vi "New GUID.vi"(8 "error in (no error)":errorcluster) -> (0 "error out":errorcluster, 2 "GUID bytes":u8[](array[numeric]) format="%02x", 3 "GUID":string)   [LabVIEW 2013]
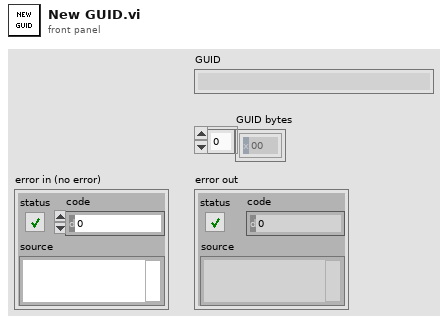
[diagram p1: front panel]
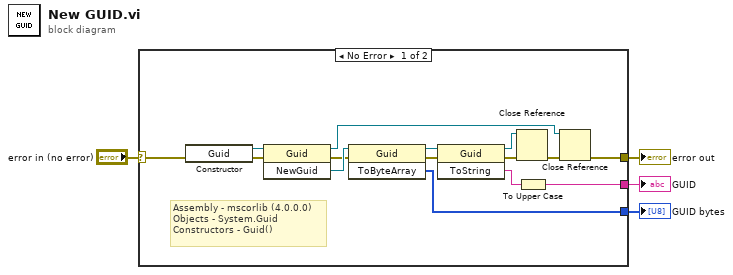
[diagram p0: block diagram]
diagram:
  n1 = case shown="No Error" "error in (no error)" {
    selector: "error in (no error)" -> [w5 w20]
    tunnel: [w9 _] -> w4
    tunnel: [w7 w20] -> w3
    tunnel: [w6 _] -> w2
    frame No Error {
      # "Assembly - mscorlib (4.0.0.0)\nObjects - System.Guid\nConstructors - Guid()"
      n2 = constructor class="Guid"(error in=w5) -> (reference out=w19:refnum<k24>, error out=w16:errorcluster)  [unwired: 2 in, 1 out]
      n3 = invoke class="Guid" method="NewGuid"(reference=w19, error in=w16) -> (reference out=w17:refnum<k24>, error out=w10:errorcluster, "NewGuid"=w15:refnum<k24>)  [unwired: 1 in]
      n4 = invoke class="Guid" method="ToByteArray"(reference=w15, error in=w10) -> (reference out=w14:refnum<k24>, error out=w13:errorcluster, "ToByteArray"=w9:u8[])  [unwired: 1 in]
      n5 = invoke class="Guid" method="ToString"(reference=w14, error in=w13) -> (reference out=w11:refnum<k24>, error out=w12:errorcluster, "ToString"=w8:string)  [unwired: 1 in]
      n6 = Close Reference(reference=w11, error in (no error)=w12) -> (error out=w18:errorcluster)
      n7 = To Upper Case(1:w8) -> (0:w6:string)
      n8 = Close Reference(reference=w17, error in (no error)=w18) -> (error out=w7:errorcluster)
    }
    frame Error {
    }
  }
  "GUID bytes" <- w4
  "GUID" <- w2
  "error out" <- w3
